vi "Connected.vi"(8 "error in (no error)":errorcluster, 11 "Connecting in":refnum<class "Connecting.lvclass">) -> (0 "error out":errorcluster, 3 "Connecting out":refnum<class "Connecting.lvclass">)   [LabVIEW 2013, in "Receiver.lvlib" / "Receive Commands Using State Actors.lvlib" / "Connect Command.lvlib" / "Executing States.lvlib" / "Connecting.lvclass"]
uses:
  Connecting.lvclass
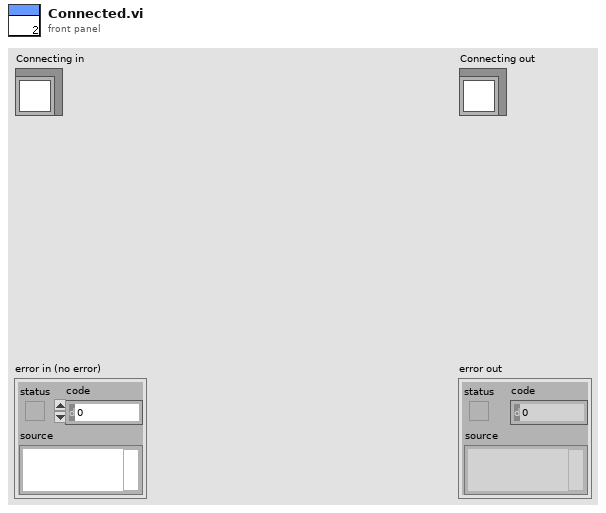
[diagram p1: front panel]
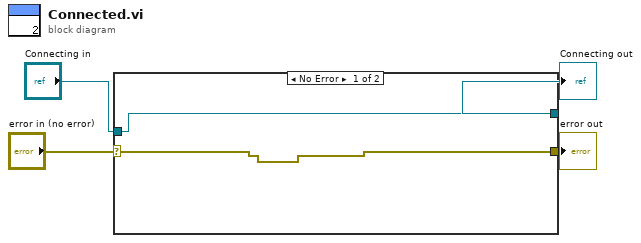
[diagram p0: block diagram]
diagram:
  n1 = case shown="No Error" "error in (no error)" {
    selector: "error in (no error)" -> [w6 w8]
    tunnel: [w6 w8] -> w3
    tunnel: [w5 w7] -> w1
    tunnel: "Connecting in" -> [w5 w7]
    frame No Error {
    }
    frame Error {
    }
  }
  "error out" <- w3
  "Connecting out" <- w1
